vi "Status Upload(Test Unit).vi"(4 "Message Queue":refnum<class "Delacor_lib_QMH_Message Queue.lvclass">, 5 "Event Data":cluster{"Status":string, "Module ID":i32}, 6 "User Event Ref":refnum<user-event>, 7 "Event Common Data":T2 {"Event Source" items=["LabVIEW UI"=0, "ActiveX"=1, "User Event"=25]}) -> ()   [LabVIEW 2025]
uses:
  <vilib>/event_ctls.llb/eventsource.ctl
  Test Unit/Status Updated Argument--cluster.ctl
  <vilib>/Delacor/Delacor QMH/Libraries/Message Queue_class/Delacor_lib_QMH_Message Queue.lvclass
  <vilib>/Delacor/Delacor QMH/Libraries/Message Queue_class/Delacor_lib_QMH_Message Queue.lvclass/Delacor_lib_QMH_Message Queue.ctl
  <vilib>/Delacor/Delacor QMH/Libraries/Message Queue_class/Delacor_lib_QMH_Enqueue Message (Single).vi
  Test Unit/Test Unit.lvlib
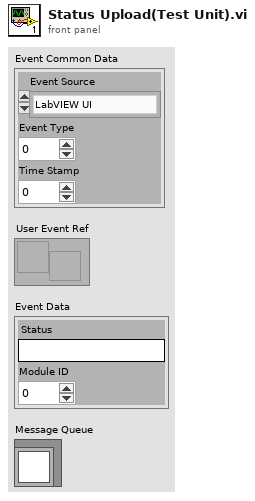
[diagram p1: front panel]
types:
  T1 = typedef "eventsource.ctl" = u32
  T2 = cluster{"Event Source":T1, "Event Type":u32, "Time Stamp":u32}
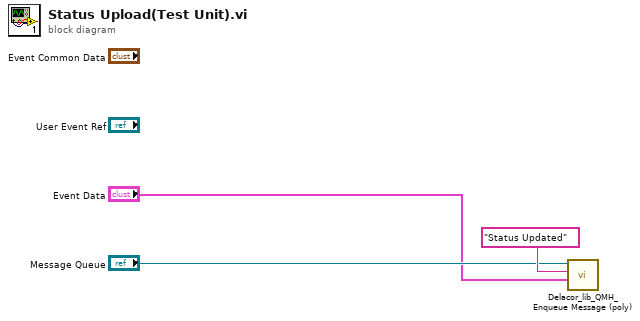
[diagram p0: block diagram]
diagram:
  n1 = call-poly <vilib>:"Delacor_lib_QMH_Enqueue Message (poly).vi"("Message Data"="Event Data", "Message"="Status Updated", "Message Queue in"="Message Queue") -> ()  [unwired: 7 in, 2 out]
